vi "Keysight_N6700C_TurnOff.vi"(2 "error in (no error)":errorcluster, 3 "VISA resource name":refnum<visa-resource-name>) -> (0 "error out":errorcluster)   [LabVIEW 2018]
uses:
  SupportVIs/Agilent N6700 Series.lvlib
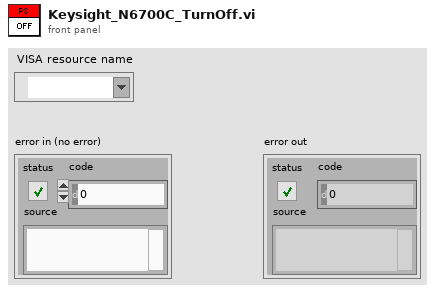
[diagram p1: front panel]
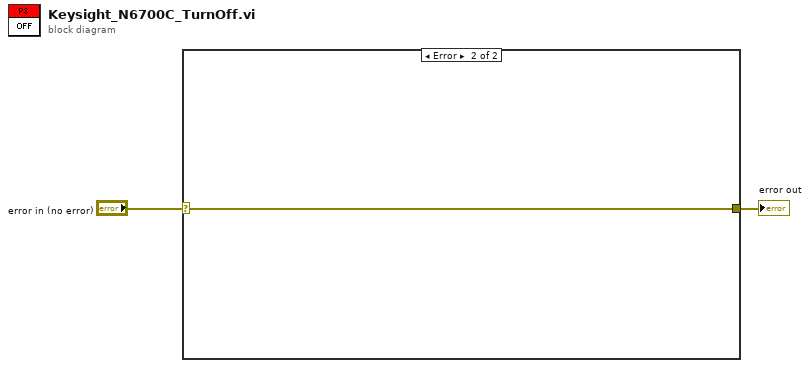
[diagram p0: block diagram]
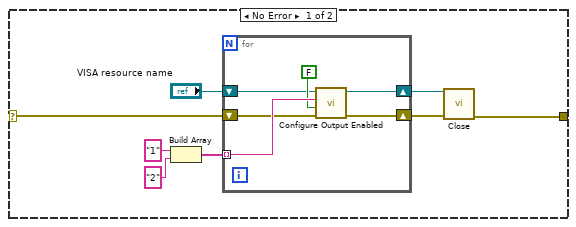
[diagram p2: hidden frame]
diagram:
  n1 = case shown="Error" "error in (no error)" {
    selector: "error in (no error)" -> [w3 w17]
    tunnel: [w5 w17] -> w2
    frame No Error {
      n2 = Build Array("1" ("Channel Name (1)"), "2" ("Channel Name (2)")) -> (w8:string[])
      n3 = for {
        tunnel: w8 -> [w16] mode=indexing
        shift-right: [w14] -> w7
        shift-left: "VISA resource name" -> [w13]
        shift-right: [w11] -> w4
        shift-left: w3 -> [w12]
        n4 = call "Configure Output Enabled.vi"("error in (no error)"=w12, "Enable Output (False)"=FALSE, "Channel Name (1)"=w16, "VISA resource name"=w13) -> ("error out"=w11:errorcluster, "VISA resource name out"=w14:refnum<visa-resource-name>)  [unwired: 6 in]
      }
      n5 = call "Close.vi"("VISA resource name"=w7, "error in (no error)"=w4) -> ("error out"=w5:errorcluster)  [unwired: 13 in]
    }
    frame Error {
    }
  }
  "error out" <- w2
